vi "getPayloadRequirement.vi"(11 "UNSUBSCRIBE in":refnum<class "UNSUBSCRIBE.lvclass">) -> (2 "Requirement":T1, 3 "UNSUBSCRIBE out":refnum<class "UNSUBSCRIBE.lvclass">)   [LabVIEW 2013, in "UNSUBSCRIBE.lvclass"]
uses:
  UNSUBSCRIBE.lvclass
  Requirement -- enum.ctl
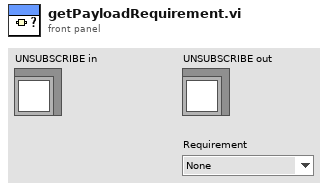
[diagram p1: front panel]
types:
  T1 = typedef "Requirement -- enum.ctl" = enum16{"None", "Optional", "Required"}
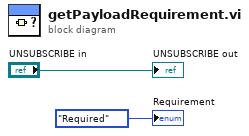
[diagram p0: block diagram]
diagram:
  "UNSUBSCRIBE out" <- "UNSUBSCRIBE in"
  "Requirement" <- Requirement_--_enum."Required" ("Requirement")
